vi "ExecuteMenu.vi"(8 "ErrorIn":errorcluster, 10 "ItemPath":string, 11 "DemoApplicationIn":refnum<class "DemoApplication.lvclass">) -> (0 "ErrorOut":errorcluster, 3 "DemoApplicationOut":refnum<class "DemoApplication.lvclass">)   [LabVIEW 2021, in "DemoApplication.lvclass"]
uses:
  DemoApplication.lvclass
  .Externals/Interface_TAF_ITAFObject/ITAFObject/ITAFObject.lvclass
  .Externals/Library_UserInterface_FrontPanelControl/FrontPanelControl/FrontPanelControl.lvclass
  .Externals/Interface_UserInterface_IFrontPanel/IFrontPanel/IFrontPanel.lvclass
  .Externals/Interface_TAF_ITextViewer/ITAFTextViewer.lvclass
  .Externals/Interface_TAF_IApplicationConfiguration/IApplicationConfiguration/IApplicationConfiguration.lvclass
  .Externals/Library_TAF_ApplicationFramework/MasterGUI/MasterGUI.lvclass
  DemoApplication.lvclass/DemoApplication.ctl
  .Externals/Library_TAF_ApplicationFramework/Application/Application.lvclass
  C:/Localdata/Projects/TriekselSoft/TriekselsoftApplicationFramework/Source/.Externals/Interface_Object_ICreateDestroy/ICreateDestroy/ICreateDestroy.lvclass
  C:/Localdata/Projects/TriekselSoft/TriekselsoftApplicationFramework/Source/IInterface/IInterface.lvclass
  C:/Localdata/Projects/TriekselSoft/TriekselsoftApplicationFramework/Source/.Externals/Interface_UserInterface_IFrontPanel/IFrontPanel/IFrontPanel.lvclass
  C:/Localdata/Projects/TriekselSoft/TriekselsoftApplicationFramework/Source/.Externals/Interface_Object_IPersistentData/IPersistentData/IPersistentData.lvclass
  C:/Localdata/Projects/TriekselSoft/TriekselsoftApplicationFramework/Source/.Externals/Interface_TAF_ITAFObject/ITAFObject/ITAFObject.lvclass
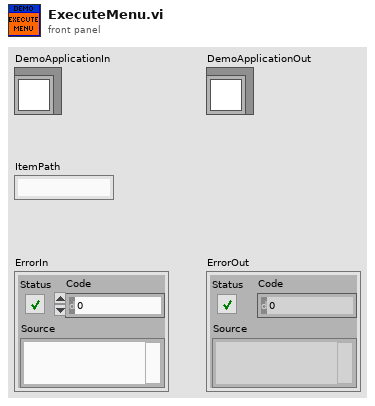
[diagram p1: front panel]
types:
  T1 = typedef "DemoApplication.lvclass/ObjectAttributes.ctl" = cluster{"Interfaces":cluster{"Authorizer":refnum<class "IAuthorization.lvclass">, "TextViewer":refnum<class "ITAFTextViewer.lvclass">, "ApplicationConfiguration":refnum<class "IApplicationConfiguration.lvclass">, "Tracer":refnum<class "IFrontPanel.lvclass">}, "Persistent":cluster{"MenuEnables":cluster{"MenuTag":string, "MenuExpression":string}[], "TextDockSubPanelName":string}}
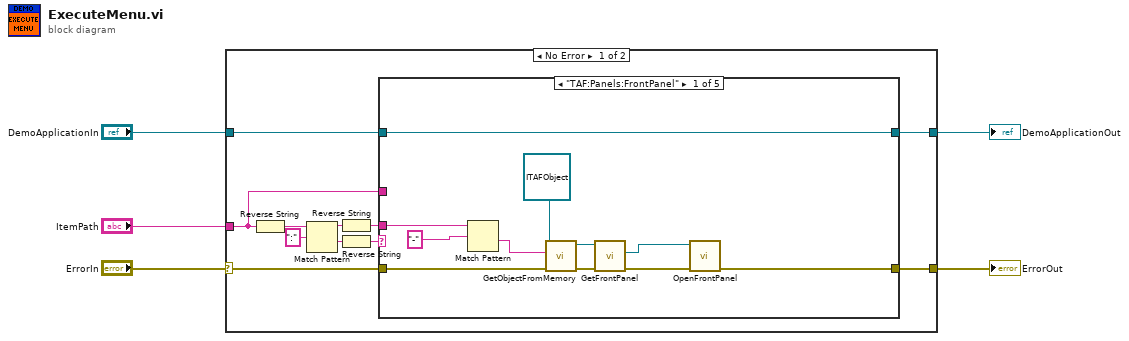
[diagram p0: block diagram]
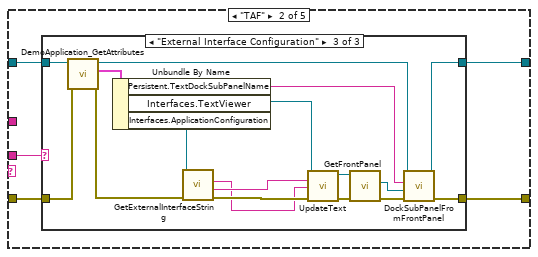
[diagram p2: hidden frame]
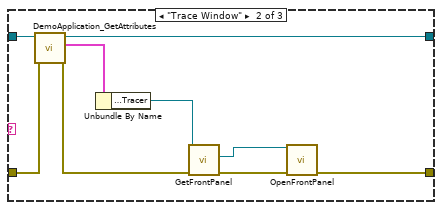
[diagram p4: hidden frame]
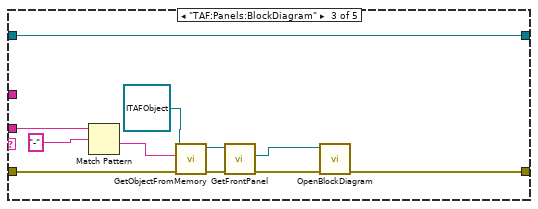
[diagram p5: hidden frame]
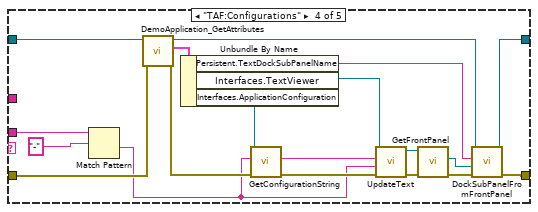
[diagram p6: hidden frame]
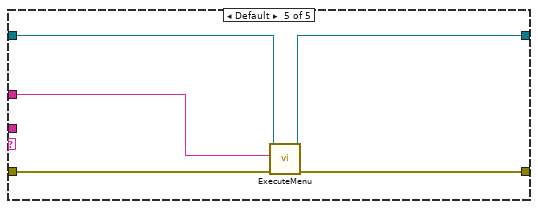
[diagram p7: hidden frame]
diagram:
  n1 = case shown="No Error" "ErrorIn" {
    selector: "ErrorIn" -> [w15 w97]
    tunnel: [w14 w96] -> w3
    tunnel: "DemoApplicationIn" -> [w13 w96]
    tunnel: [w16 w97] -> w5
    tunnel: "ItemPath" -> [w6 _]
    frame No Error {
      n2 = Reverse String(1:w6) -> (0:w10:string)
      n3 = Match Pattern(string=w10, regular expression=":") -> (before substring=w8:string, after substring=w9:string)  [unwired: 1 in, 2 out]
      n4 = Reverse String(1:w8) -> (0:w11:string)
      n5 = Reverse String(1:w9) -> (0:w12:string)
      n6 = case shown="\"TAF:Panels:FrontPanel\"" w12 {
        tunnel: w11 -> [w19 w28 w63 w83 _]
        tunnel: [w25 w32 w69 w85 w94] -> w16
        tunnel: w15 -> [w24 w31 w68 w89 w95]
        tunnel: [w17 w29 w64 w76 w92] -> w14
        tunnel: w13 -> [w17 w30 w64 w84 w93]
        tunnel: w6 -> [_ _ _ _ w91]
        frame "TAF:Panels:FrontPanel" {
          n7 = Match Pattern(string=w19, regular expression="-") -> (after substring=w18:string)  [unwired: 1 in, 3 out]
          n8 = call "GetObjectFromMemory.vi"("ErrorIn"=w24, "ObjectName"=w18, "Type"=refnum<class "ITAFObject.lvclass"> refnum ("NamedCreator")) -> ("ErrorOut"=w27:errorcluster, "ObjectOut"=w22:refnum<class "ITAFObject.lvclass">)  [unwired: 7 in]
          n9 = call-dynamic "GetFrontPanel.vi"("ErrorIn"=w27, "ObjectIn"=w22) -> ("ErrorOut"=w26:errorcluster, "FrontPanelControl"=w21:refnum<class "FrontPanelControl.lvclass">)  [unwired: 7 in, 1 out]
          n10 = call-dynamic "OpenFrontPanel.vi"("ErrorIn"=w26, "ObjectIn"=w21) -> ("ErrorOut"=w25:errorcluster)  [unwired: 8 in, 1 out]
        }
        frame "TAF" {
          n11 = case shown="\"External Interface Configuration\"" w28 {
            tunnel: [w34 w43 w55] -> w32
            tunnel: w30 -> [w33 w39 w54]
            tunnel: [w33 w38 w44] -> w29
            tunnel: w31 -> [w34 w42 w60]
            frame Default {
            }
            frame "Trace Window" {
              n12 = call "DemoApplication_GetAttributes.vi"("error in (no error)"=w42, "reference in"=w39) -> ("error out"=w40:errorcluster, "Data"=w37:T1, "reference out"=w38:refnum<class "DemoApplication.lvclass">)  [unwired: 6 in, 1 out]
              n13 = Unbundle By Name(w37) -> ("Interfaces.Tracer"=w35:refnum<class "IFrontPanel.lvclass">)
              n14 = call-dynamic "GetFrontPanel.vi"("ErrorIn"=w40, "ObjectIn"=w35) -> ("ErrorOut"=w41:errorcluster, "FrontPanelControl"=w36:refnum<class "FrontPanelControl.lvclass">)  [unwired: 7 in, 1 out]
              n15 = call-dynamic "OpenFrontPanel.vi"("ErrorIn"=w41, "ObjectIn"=w36) -> ("ErrorOut"=w43:errorcluster)  [unwired: 8 in, 1 out]
            }
            frame "External Interface Configuration" {
              n16 = call "DemoApplication_GetAttributes.vi"("error in (no error)"=w60, "reference in"=w54) -> ("error out"=w56:errorcluster, "Data"=w46:T1, "reference out"=w45:refnum<class "DemoApplication.lvclass">)  [unwired: 6 in, 1 out]
              n17 = Unbundle By Name(w46) -> ("Persistent.TextDockSubPanelName"=w47:string, "Interfaces.TextViewer"=w52:refnum<class "ITAFTextViewer.lvclass">, "Interfaces.ApplicationConfiguration"=w50:refnum<class "IApplicationConfiguration.lvclass">)
              n18 = call-dynamic "GetExternalInterfaceString.vi"("ErrorIn"=w56, "ReferenceIn"=w50) -> ("ErrorOut"=w58:errorcluster, "String"=w53:string, "Identification"=w49:string)  [unwired: 6 in, 1 out]
              n19 = call-dynamic "UpdateText.vi"("ErrorIn"=w58, "ID"=w49, "Text"=w53, "ObjectIn"=w52) -> ("ErrorOut"=w59:errorcluster, "ObjectOut"=w51:refnum<class "ITAFTextViewer.lvclass">)  [unwired: 6 in]
              n20 = call-dynamic "GetFrontPanel.vi"("ErrorIn"=w59, "ObjectIn"=w51) -> ("ErrorOut"=w57:errorcluster, "FrontPanelControl"=w48:refnum<class "FrontPanelControl.lvclass">)  [unwired: 7 in, 1 out]
              n21 = call-dynamic "DockSubPanelFromFrontPanel.vi"("ErrorIn"=w57, "FrontPanel"=w48, "PanelLabel"=w47, "ReferenceIn"=w45) -> ("ErrorOut"=w55:errorcluster, "ReferenceIn"=w44:refnum<class "DemoApplication.lvclass">)  [unwired: 6 in]
            }
          }
        }
        frame "TAF:Panels:BlockDiagram" {
          n22 = Match Pattern(string=w63, regular expression="-") -> (after substring=w61:string)  [unwired: 1 in, 3 out]
          n23 = call "GetObjectFromMemory.vi"("ErrorIn"=w68, "ObjectName"=w61, "Type"=refnum<class "ITAFObject.lvclass"> refnum ("NamedCreator")) -> ("ErrorOut"=w71:errorcluster, "ObjectOut"=w66:refnum<class "ITAFObject.lvclass">)  [unwired: 7 in]
          n24 = call-dynamic "GetFrontPanel.vi"("ErrorIn"=w71, "ObjectIn"=w66) -> ("ErrorOut"=w70:errorcluster, "FrontPanelControl"=w65:refnum<class "FrontPanelControl.lvclass">)  [unwired: 7 in, 1 out]
          n25 = call-dynamic "OpenBlockDiagram.vi"("ErrorIn"=w70, "ObjectIn"=w65) -> ("ErrorOut"=w69:errorcluster)  [unwired: 8 in, 1 out]
        }
        frame "TAF:Configurations" {
          n26 = Match Pattern(string=w83, regular expression="-") -> (after substring=w72:string)  [unwired: 1 in, 3 out]
          n27 = call "DemoApplication_GetAttributes.vi"("error in (no error)"=w89, "reference in"=w84) -> ("error out"=w88:errorcluster, "Data"=w81:T1, "reference out"=w77:refnum<class "DemoApplication.lvclass">)  [unwired: 6 in, 1 out]
          n28 = Unbundle By Name(w81) -> ("Persistent.TextDockSubPanelName"=w74:string, "Interfaces.TextViewer"=w80:refnum<class "ITAFTextViewer.lvclass">, "Interfaces.ApplicationConfiguration"=w78:refnum<class "IApplicationConfiguration.lvclass">)
          n29 = call-dynamic "GetConfigurationString.vi"("ErrorIn"=w88, "Identification"=w72, "ReferenceIn"=w78) -> ("ErrorOut"=w87:errorcluster, "String"=w73:string)  [unwired: 6 in, 1 out]
          n30 = call-dynamic "UpdateText.vi"("ErrorIn"=w87, "ID"=w72, "Text"=w73, "ObjectIn"=w80) -> ("ErrorOut"=w90:errorcluster, "ObjectOut"=w79:refnum<class "ITAFTextViewer.lvclass">)  [unwired: 6 in]
          n31 = call-dynamic "GetFrontPanel.vi"("ErrorIn"=w90, "ObjectIn"=w79) -> ("ErrorOut"=w86:errorcluster, "FrontPanelControl"=w75:refnum<class "FrontPanelControl.lvclass">)  [unwired: 7 in, 1 out]
          n32 = call-dynamic "DockSubPanelFromFrontPanel.vi"("ErrorIn"=w86, "FrontPanel"=w75, "PanelLabel"=w74, "ReferenceIn"=w77) -> ("ErrorOut"=w85:errorcluster, "ReferenceIn"=w76:refnum<class "DemoApplication.lvclass">)  [unwired: 6 in]
        }
        frame Default {
          n33 = call-parent "ExecuteMenu.vi"("ErrorIn"=w95, "ItemPath"=w91, "MasterGUIIn"=w93) -> ("ErrorOut"=w94:errorcluster, "MasterGUIOut"=w92:refnum<class "DemoApplication.lvclass">)  [unwired: 7 in]
        }
      }
    }
    frame Error {
    }
  }
  "DemoApplicationOut" <- w3
  "ErrorOut" <- w5
